vi "Load and Unflatten Class Data.vi"(8 "error in":errorcluster, 11 "Loopback in":refnum<class "Loopback.lvclass">) -> (0 "error out":errorcluster, 3 "Loopback out":refnum<class "Loopback.lvclass">)   [LabVIEW 2020, in "Loopback.lvclass"]
uses:
  Loopback.lvclass
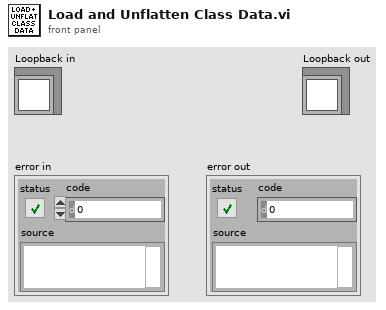
[diagram p1: front panel]
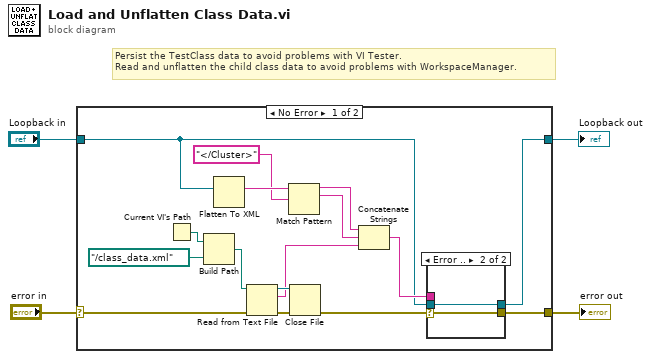
[diagram p0: block diagram]
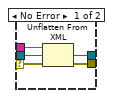
[diagram p2: hidden frame]
diagram:
  # "Persist the TestClass data to avoid problems with VI Tester.\nRead and unflatten the child class data to avoid problems with WorkspaceManager."
  n1 = case shown="No Error" "error in" {
    selector: "error in" -> [w18 w28]
    tunnel: [w14 w28] -> w3
    tunnel: "Loopback in" -> [w10 w29]
    tunnel: [w8 w29] -> w1
    frame No Error {
      n2 = Current VI's Path() -> (path=w19:path)
      n3 = Build Path(base path=w19, name or relative path=path "../class_data.xml") -> (appended path=w17:path)
      n4 = Flatten To XML(6:w10) -> (2:w13:string)
      n5 = Read from Text File(file (use dialog)=w17, error in=w18) -> (refnum out=w15:refnum<file>, text=w5:string, error out=w16:errorcluster)  [unwired: 2 in, 1 out]
      n6 = Match Pattern(string=w13, regular expression="</Cluster>") -> (before substring=w12:string, match substring=w9:string)  [unwired: 1 in, 2 out]
      n7 = Close File(refnum=w15, error in=w16) -> (error out=w7:errorcluster)  [unwired: 1 out]
      n8 = Concatenate Strings(w12, w9, w5) -> (w11:string)
      n9 = case shown="Error .." w7 {
        selector: w7 -> [w21 w27]
        tunnel: [w25 w27] -> w14
        tunnel: w11 -> [w24 _]
        tunnel: w10 -> [w23 w26]
        tunnel: [w22 w26] -> w8
        frame No Error {
          n10 = Unflatten From XML(xml string=w24, type=w23, error in (no error)=w21) -> (value=w22:refnum<class "Loopback.lvclass">, error out=w25:errorcluster)
        }
        frame Error {
        }
      }
    }
    frame Error {
    }
  }
  "error out" <- w3
  "Loopback out" <- w1
